vi "Check Response from Set Command.vi"(8 "error in (no error)":errorcluster, 10 "Command":string, 11 "Response":string) -> (0 "error out":errorcluster, 1 "Error":bool, 2 "NACK":bool, 3 "ACK":bool)   [LabVIEW 2021, in "Environment Chamber.lvlib" / "Climatic Chamber.lvlib"]
uses:
  Climatic Chamber.lvlib
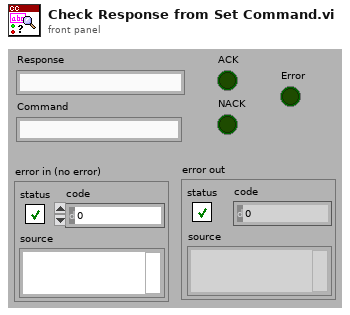
[diagram p1: front panel]
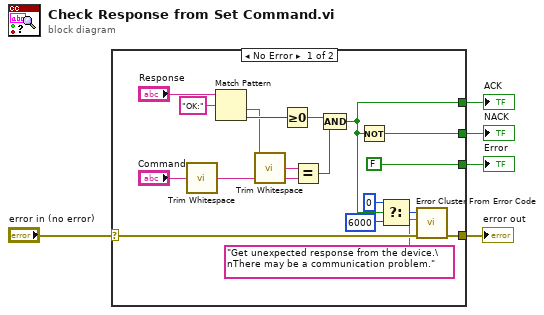
[diagram p0: block diagram]
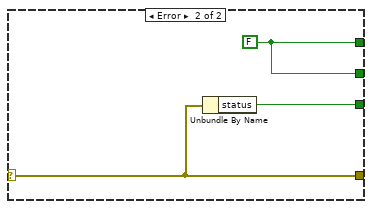
[diagram p2: hidden frame]
diagram:
  n1 = case shown="No Error" "error in (no error)" {
    selector: "error in (no error)" -> [w23 w26]
    tunnel: [w11 w26] -> w4
    tunnel: [FALSE ("status") w25] -> w3
    tunnel: [w7 w24] -> w2
    tunnel: [w18 w24] -> w1
    frame No Error {
      n2 = call <vilib>:"Trim Whitespace.vi"("string"="Command") -> ("trimmed string"=w14:string)  [unwired: 1 in]
      n3 = Match Pattern(string="Response", regular expression="OK:") -> (after substring=w16:string, offset past match=w20:i32)  [unwired: 1 in, 2 out]
      n4 = call <vilib>:"Trim Whitespace.vi"("string"=w16) -> ("trimmed string"=w15:string)  [unwired: 1 in]
      n5 = Greater Or Equal To 0?(x=w20) -> (x >= 0?=w19:bool)
      n6 = Equal?(x=w15, y=w14) -> (x = y?=w13:bool)
      n7 = Compound Arithmetic op=AND(w19, w13) -> (w7:bool)
      n8 = Not(x=w7) -> (.not. x?=w18:bool)
      n9 = Select(t=0, s=w7, f=6000) -> (s? t:f=w10:i32)
      n10 = call <vilib>:"Error Cluster From Error Code.vi"("error in (no error)"=w23, "error message (\"\")"="Get unexpected response from the device.\nThere may be a communication problem." ("error message (\"\")"), "error code (0)"=w10) -> ("error out"=w11:errorcluster)  [unwired: 6 in]
    }
    frame Error {
      w24 = FALSE
      n11 = Unbundle By Name(w26) -> ("status"=w25:bool)
    }
  }
  "error out" <- w4
  "ACK" <- w2
  "NACK" <- w1
  "Error" <- w3
